vi "ALL_FILTER.vi"() -> ()   [LabVIEW 2020]
uses:
  <vilib>/Analysis/3filter.llb/Savitzky-Golay Filter (DBL).vi
  <vilib>/Analysis/3filter.llb/Zero Phase Filter (DBL).vi
  <vilib>/Analysis/NI_AALBase.lvlib
  <vilib>/Analysis/NI_AALPro.lvlib
  <vilib>/Analysis/2dsp.llb/1D Convolution (DBL).vi
panel:
  out "Channel 2":waveform(dbl)(graph)
  out "Find Best Filter":waveform(dbl)[](graph)
  in  "half-width":i32=5
  in  "rank":i32=2
  in  "polynomial order":i32=3
  in  "side points":i32=6
  out "ALL FILTER":waveform(dbl)[](graph)
  in  "Lower Cut-Off Frequency":dbl=100.0 caption="Lower Cut-Off"
  out "Channel 3":waveform(dbl)(graph)
  out "Channel 1":waveform(dbl)(graph)
  in  "file path (IN)":path
  out "Waveform Graph":waveform(dbl)[](graph)
  # "Zero Phase Moving Avg -Rectangular"
  # "Zero Phase Moving Avg -Triangular"
  # "Rectangle-Moving Average 4-HalfWidth"
  # "Triangle-Moving Average 4-HalfWidth"
  # "Low-Pass Filter"
  # "(ICE)"
  # "(VGE)"
  # "Savizky-Golay Filter"
  # "Zero Phase Filter with Smoothing Coeff"
  # "Median Filter"
  # "Low Pass Filter"
  # "(VCE)"
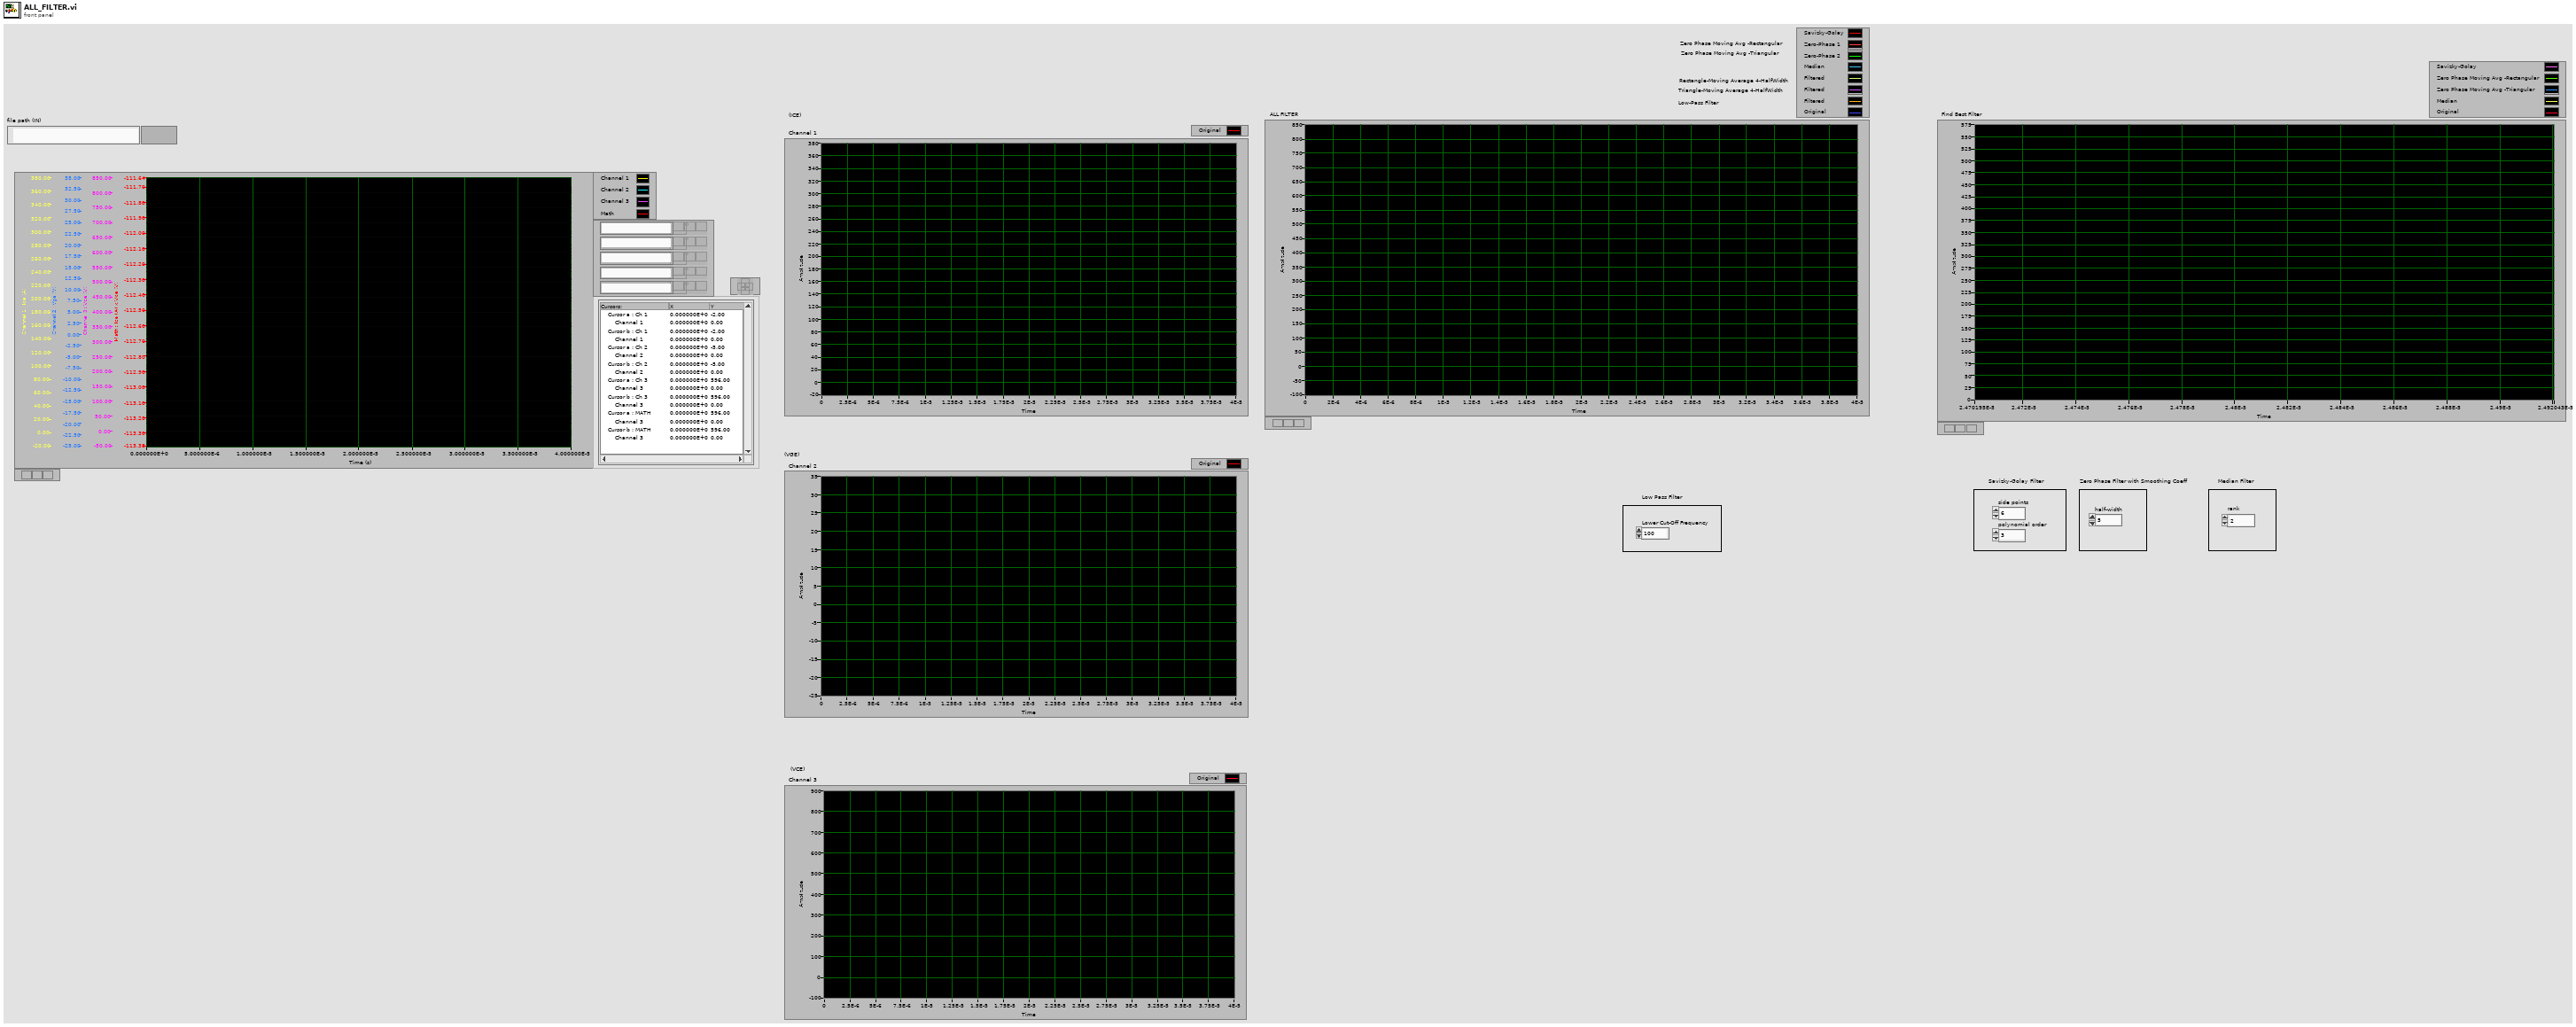
[diagram p1: front panel]
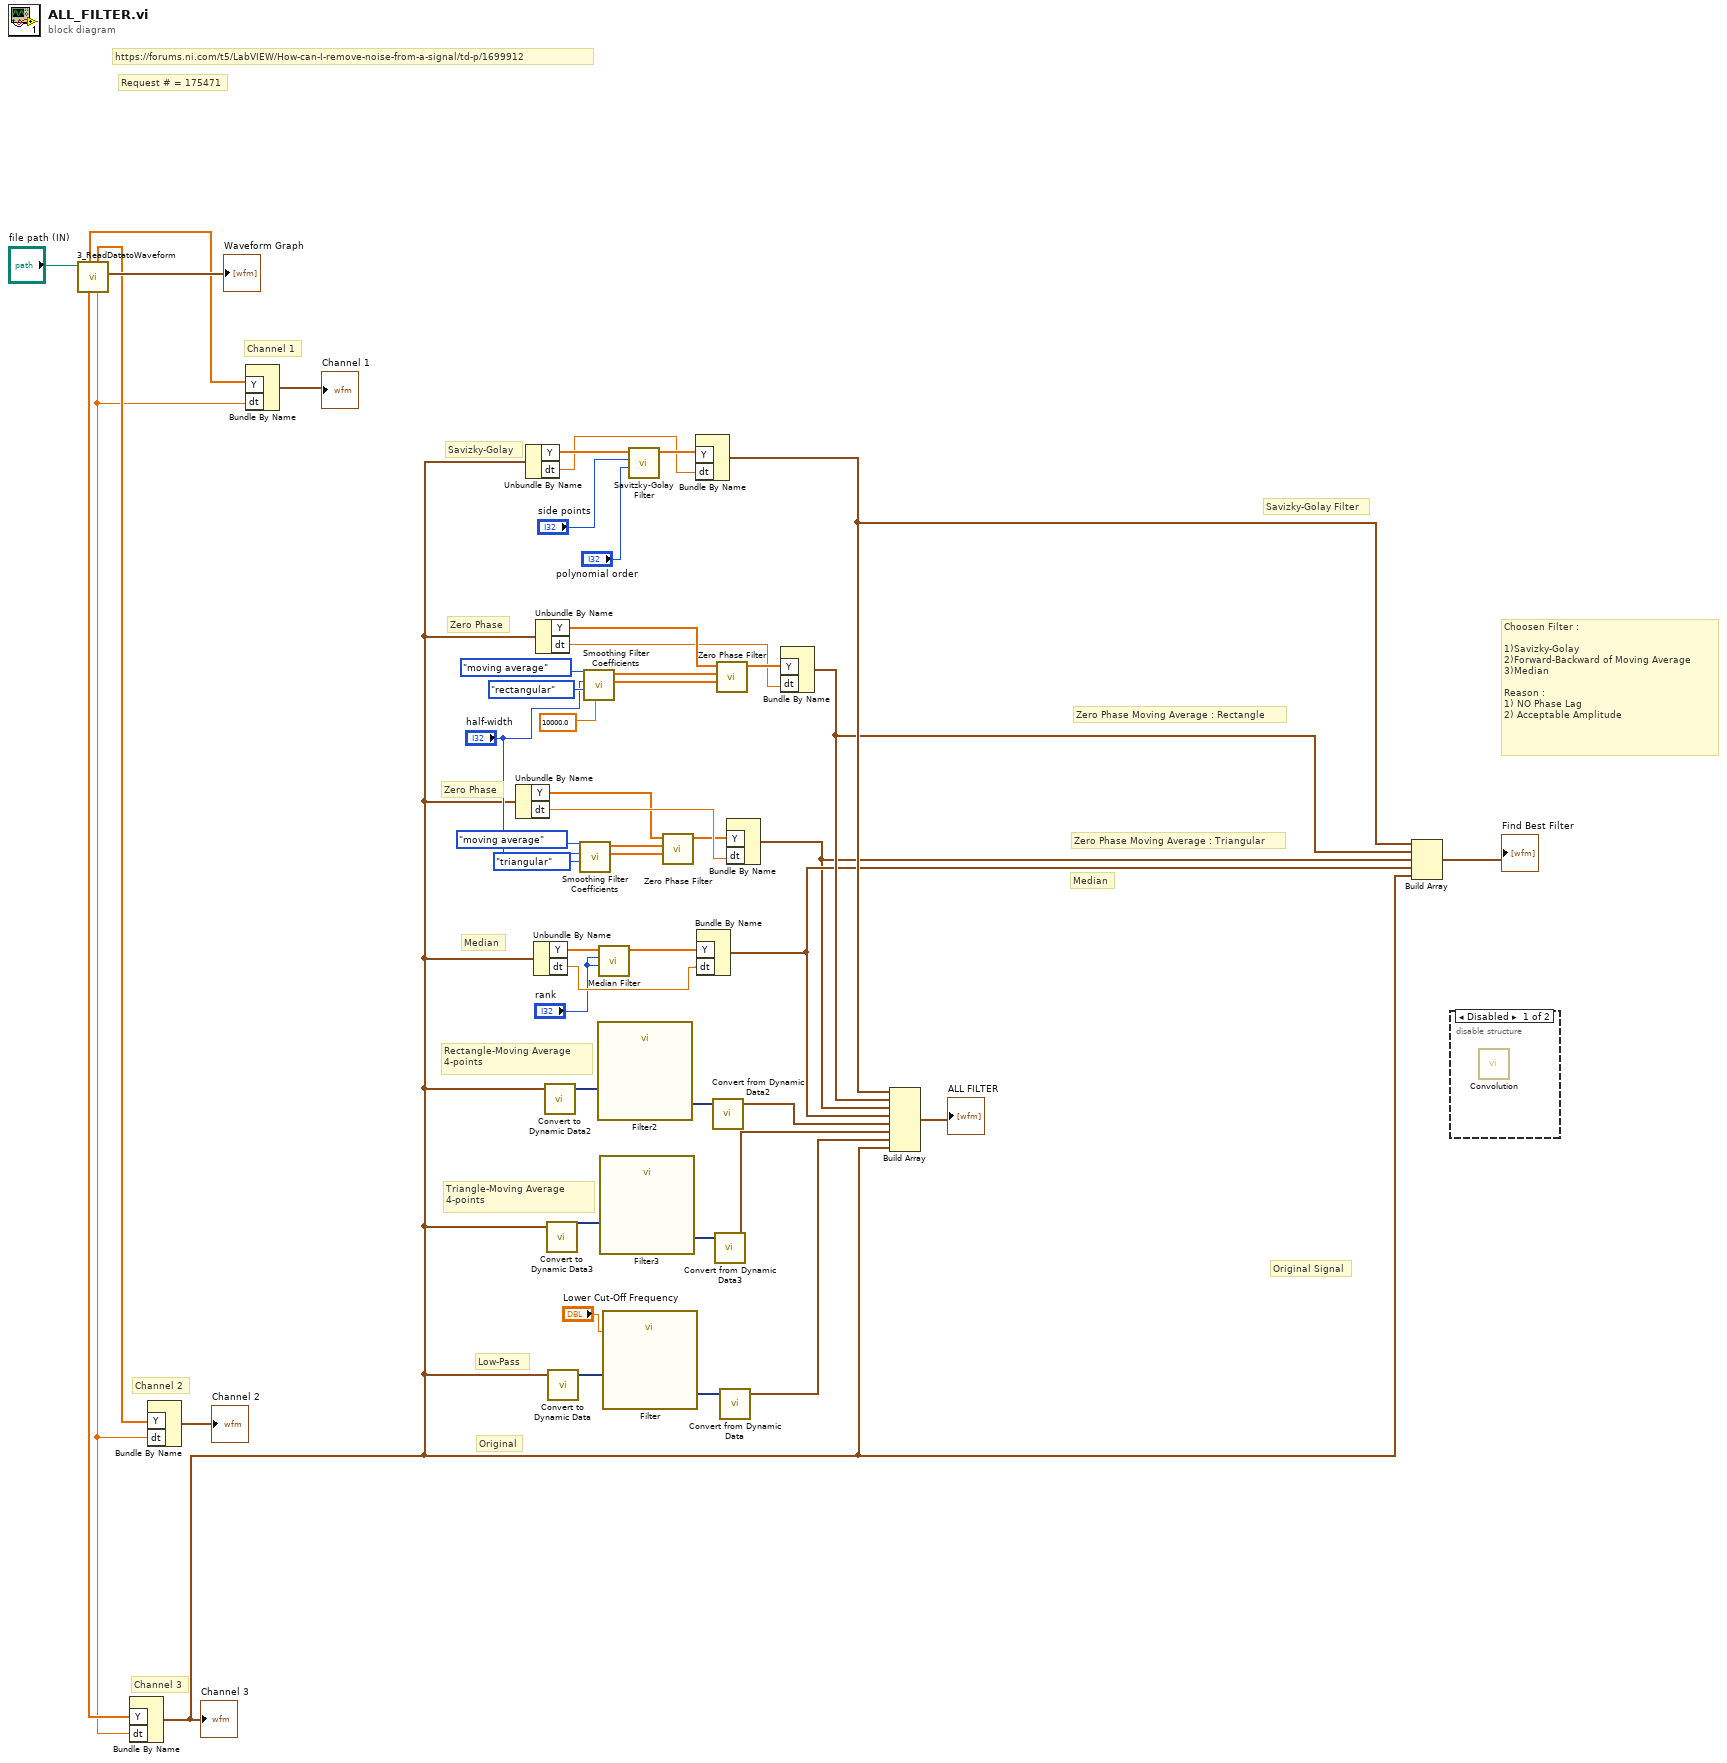
[diagram p0: block diagram]
diagram:
  # "Zero Phase Moving Average : Triangular"
  # "Zero Phase"
  # "Median"
  # "Zero Phase Moving Average : Rectangle"
  # "Savizky-Golay Filter"
  # "Original Signal"
  # "Choosen Filter : \n\n1)Savizky-Golay\n2)Forward-Backward of Moving Average\n3)Median\n\nReason : \n1) NO Phase Lag\n2) Acceptable Amplitude"
  # "Triangle-Moving Average\n4-points"
  # "Savizky-Golay"
  # "Request # = 175471"
  # "Zero Phase"
  # "Median"
  # "Rectangle-Moving Average\n4-points"
  # "Low-Pass"
  # "Original"
  # "Channel 3"
  # "Channel 2"
  # "Channel 1"
  # "https://forums.ni.com/t5/LabVIEW/How-can-I-remove-noise-from-a-signal/td-p/1699912"
  n1 = call "3_ReadDatatoWaveform.vi"("file path (IN)"="file path (IN)") -> ("Waveform Graph"=→"Waveform Graph":waveform(dbl)[], "dt"=w46:dbl, "Ch 2 Data"=w48:dbl[], "Ch 3 Data"=w47:dbl[], "Ch 1 Data"=w49:dbl[])  [unwired: 4 in, 2 out]
  n2 = Bundle By Name("Y"=w47, "dt"=w46) -> (w1:waveform(dbl))  [unwired: 1 in]
  "Channel 3" <- w1
  n3 = Bundle By Name("Y"=w48, "dt"=w46) -> (→"Channel 2":waveform(dbl))  [unwired: 1 in]
  n4 = Bundle By Name("Y"=w49, "dt"=w46) -> (→"Channel 1":waveform(dbl))  [unwired: 1 in]
  n5 = Unbundle By Name(w1) -> ("Y"=w6:dbl[], "dt"=w8:dbl)
  n6 = Unbundle By Name(w1) -> ("Y"=w33:dbl[], "dt"=w31:dbl)
  n7 = Unbundle By Name(w1) -> ("Y"=w39:dbl[], "dt"=w37:dbl)
  n8 = Unbundle By Name(w1) -> ("Y"=w36:dbl[], "dt"=w34:dbl)
  n9 = call "Convert to Dynamic Data2"("Waveform"=w1) -> ("Dynamic Data Type"=w41:dynamicdata)  [unwired: 3 in]
  n10 = call "Convert to Dynamic Data3"("Waveform"=w1) -> ("Dynamic Data Type"=w29:dynamicdata)  [unwired: 3 in]
  n11 = call "Convert to Dynamic Data"("Waveform"=w1) -> ("Dynamic Data Type"=w42:dynamicdata)  [unwired: 3 in]
  n12 = call <vilib>:"Smoothing Filter Coefficients.vi"("shape"=enum16{"rectangular", "triangular"}."triangular", "half-width"="half-width", "type"=enum16{"moving average", "exponential"}."moving average") -> ("forward coefficients"=w11:dbl[], "reverse coefficients"=w12:dbl[])  [unwired: 6 in, 1 out]
  n13 = call <vilib>:"Smoothing Filter Coefficients.vi"("fs"=10000.0 ("sampling freq: fs"), "shape"=enum16{"rectangular", "triangular"}."rectangular", "half-width"="half-width", "type"=enum16{"moving average", "exponential"}."moving average") -> ("forward coefficients"=w21:dbl[], "reverse coefficients"=w20:dbl[])  [unwired: 5 in, 1 out]
  n14 = call "Filter2"("Signal"=w41) -> ("Filtered Signal"=w40:dynamicdata)  [unwired: 9 in, 1 out]
  n15 = call <vilib>:"Median Filter.vi"("right rank"="rank", "left rank"="rank", "X"=w39) -> ("Filtered X"=w38:dbl[])  [unwired: 7 in, 1 out]
  n16 = call "Filter3"("Signal"=w29) -> ("Filtered Signal"=w30:dynamicdata)  [unwired: 9 in, 1 out]
  n17 = call "Filter"("Lower Cut-Off"="Lower Cut-Off Frequency", "Signal"=w42) -> ("Filtered Signal"=w43:dynamicdata)  [unwired: 8 in, 1 out]
  n18 = call-poly <vilib>:"Savitzky-Golay Filter.vi"("polynomial order"="polynomial order", "side points"="side points", "X"=w33) -> ("Filtered X"=w32:dbl[])  [unwired: 7 in, 1 out]
  n19 = call-poly <vilib>:"Zero Phase Filter.vi"("Forward Coefficients"=w11, "Reverse Coefficients"=w12, "X"=w6) -> ("Filtered X"=w7:dbl[])  [unwired: 7 in, 1 out]
  n20 = Bundle By Name("Y"=w32, "dt"=w31) -> (w18:waveform(dbl))  [unwired: 1 in]
  n21 = Bundle By Name("Y"=w38, "dt"=w37) -> (w13:waveform(dbl))  [unwired: 1 in]
  n22 = call "Convert from Dynamic Data2"("Dynamic Data Type"=w40) -> ("Waveform"=w14:waveform(dbl))  [unwired: 3 in]
  n23 = call "Convert from Dynamic Data3"("Dynamic Data Type"=w30) -> ("Waveform"=w15:waveform(dbl))  [unwired: 3 in]
  n24 = call-poly <vilib>:"Zero Phase Filter.vi"("Forward Coefficients"=w21, "Reverse Coefficients"=w20, "X"=w36) -> ("Filtered X"=w35:dbl[])  [unwired: 7 in, 1 out]
  n25 = call "Convert from Dynamic Data"("Dynamic Data Type"=w43) -> ("Waveform"=w16:waveform(dbl))  [unwired: 3 in]
  n26 = Bundle By Name("Y"=w7, "dt"=w8) -> (w4:waveform(dbl))  [unwired: 1 in]
  n27 = Bundle By Name("Y"=w35, "dt"=w34) -> (w17:waveform(dbl))  [unwired: 1 in]
  n28 = Build Array(w18, w17, w4, w13, w14, w15, w16, w1) -> (→"ALL FILTER":waveform(dbl)[])
  n29 = Build Array(w18, w17, w4, w13, w1) -> (→"Find Best Filter":waveform(dbl)[])
  n30 = disable-structure shown="Disabled" {
    frame Disabled {
      n31 = call-poly <vilib>:"Convolution.vi"() -> ()  [unwired: 10 in, 2 out]
    }
    frame Enabled {
    }
  }
